vi "MyCreateVisaFromIP (SubVI).vi"(10 "Port":i32=33576, 11 "IP address":string="192.168.0.107") -> (3 "VISA Refnum out":refnum<visa-resource-name>)   [LabVIEW 2025, in "MyTriton.lvlib"]
uses:
  MyTriton.lvlib
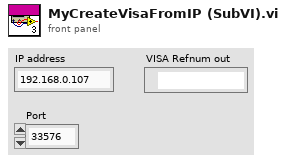
[diagram p1: front panel]
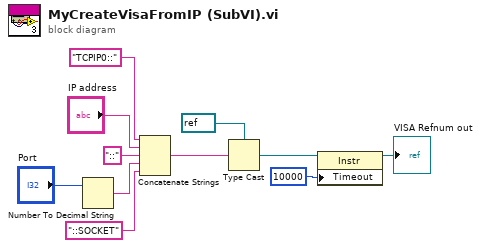
[diagram p0: block diagram]
diagram:
  n1 = Number To Decimal String(number="Port") -> (decimal integer string=w6:string)  [unwired: 1 in]
  n2 = Concatenate Strings("TCPIP0::" ("string"), "IP address", "::" ("string"), w6, "::SOCKET" ("string")) -> (w4:string)
  n3 = Type Cast(type=refnum<visa-resource-name> refnum ("VISA resource name"), x=w4) -> (*(type *) &x=w3:refnum<visa-resource-name>)
  n4 = property class="Instr"(reference=w3, "Timeout"=u32 10000 ("General Settings:Timeout Value")) -> (reference out=→"VISA Refnum out":refnum<visa-resource-name>)  [unwired: 1 in, 1 out]
